vi "labview project submission.vi"() -> ()   [LabVIEW 2012]
uses:
  <vilib>/DAQmx/read.llb/DAQmx Read (Counter DBL 1Chan 1Samp).vi
  <vilib>/DAQmx/write.llb/DAQmx Write (Analog DBL 1Chan 1Samp).vi
  <vilib>/DAQmx/write.llb/DAQmx Write (Digital U8 1Chan 1Samp).vi
  <vilib>/DAQmx/write.llb/DAQmx Write (Digital 1D Bool NChan 1Samp 1Line).vi
  <vilib>/DAQmx/read.llb/DAQmx Read (Analog DBL 1Chan 1Samp).vi
  <vilib>/DAQmx/create/channels.llb/DAQmx Create Channel (CI-Count Edges).vi
  <vilib>/DAQmx/create/channels.llb/DAQmx Create Channel (DO-Digital Output).vi
  <vilib>/DAQmx/create/channels.llb/DAQmx Create Channel (AI-Voltage-Basic).vi
  <vilib>/DAQmx/create/channels.llb/DAQmx Create Channel (AO-Voltage-Basic).vi
  <vilib>/DAQmx/miscellaneous.llb/DAQmx Fill In Error Info.vi
  KERNEL32.DLL
panel:
  out "led 3":bool
  out "led 1":bool
  out "led 2":bool
  out "7 Segment":picture
  out "Voltage:":dbl
  out "Slot Count:":dbl
  out "Data to Write":u32=255 caption="Data to Write:" format="%x"
  out "Motor:":bool[](array[boolean])
  out "Time:":string
  out "Date:":string
  in  "Dignostic":bool
  in  "?":bool
  # "Lighthouse Monitoring & Control System"
  # "Normal Mode"
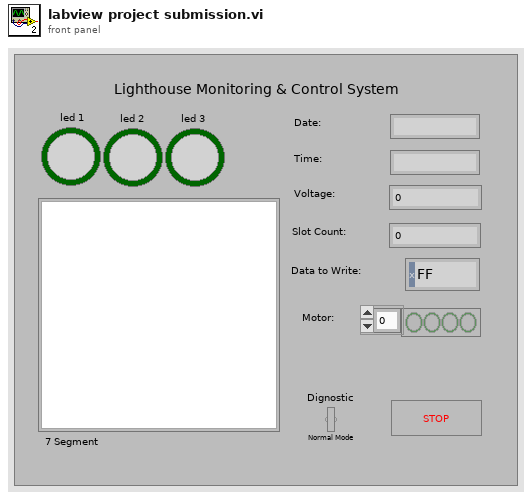
[diagram p1: front panel]
types:
  T1 = typedef "imagedata.ctl" = cluster{"image type":i32, "image depth":i32, "image":u8[], "mask":u8[], "colors":u32[], "Rectangle":cluster{"left":i16, "top":i16, "right":i16, "bottom":i16}}
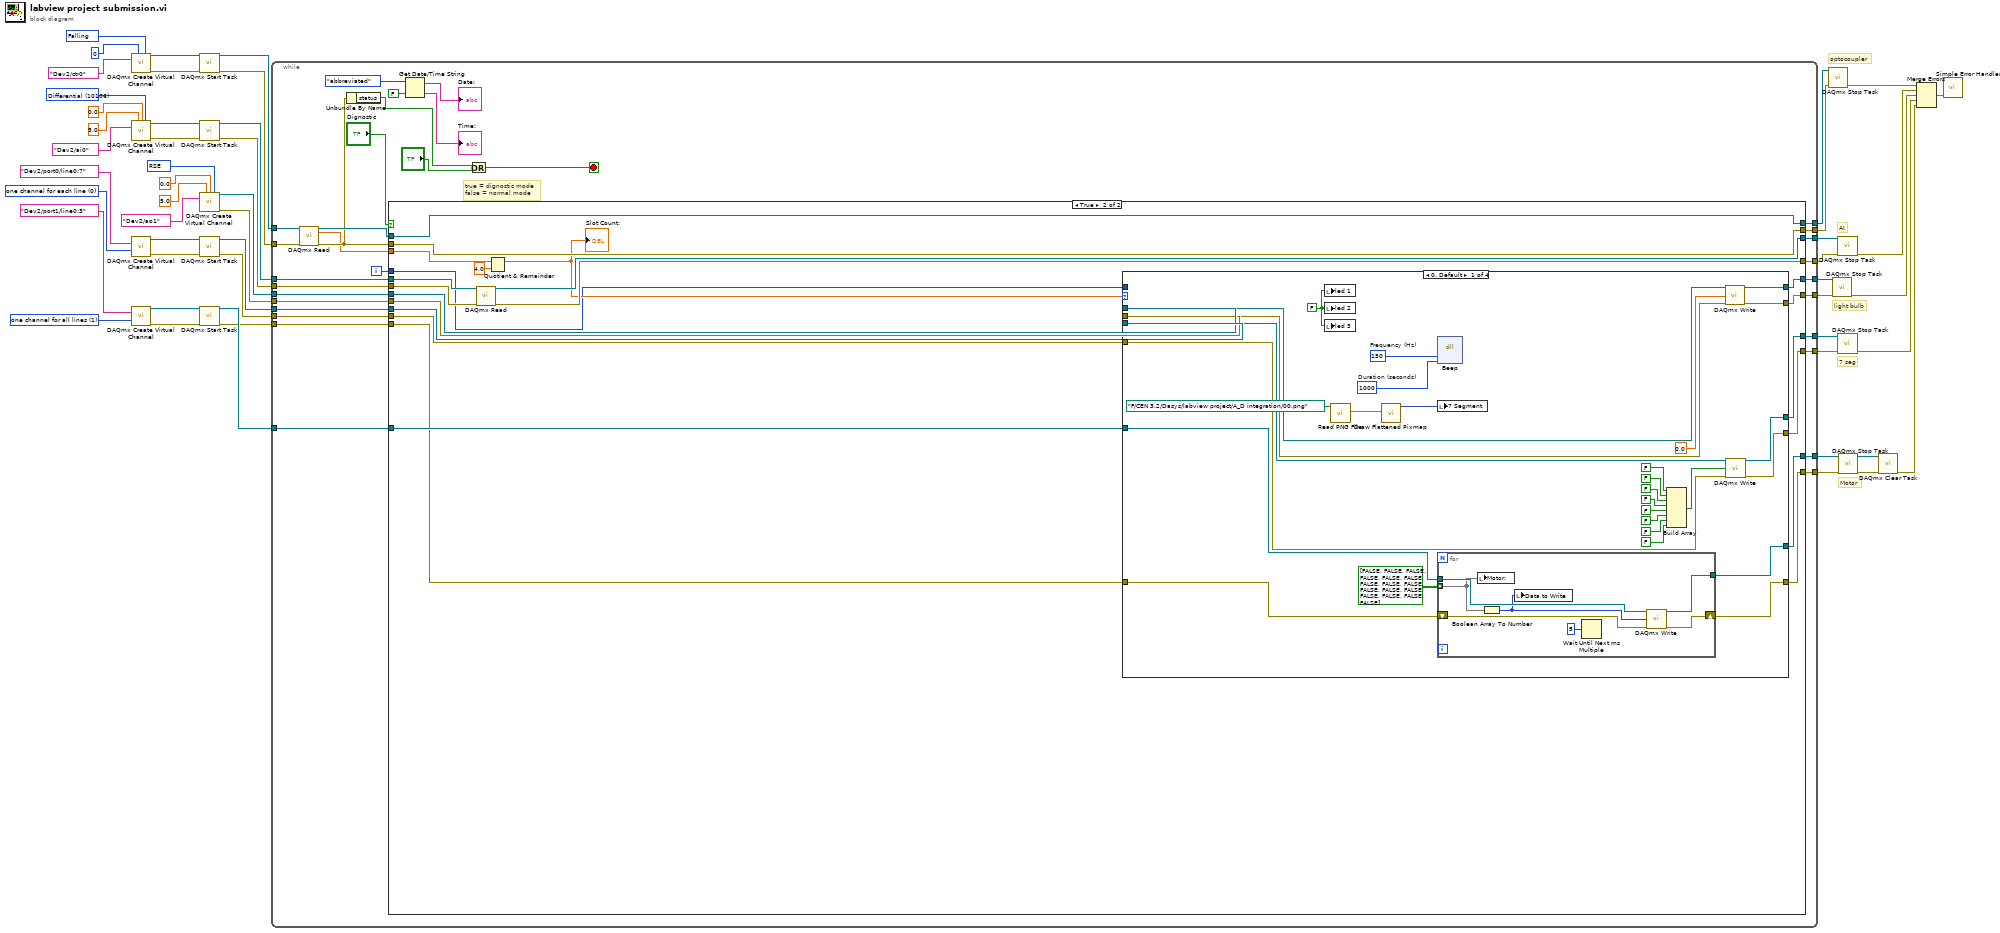
[diagram p0: block diagram]
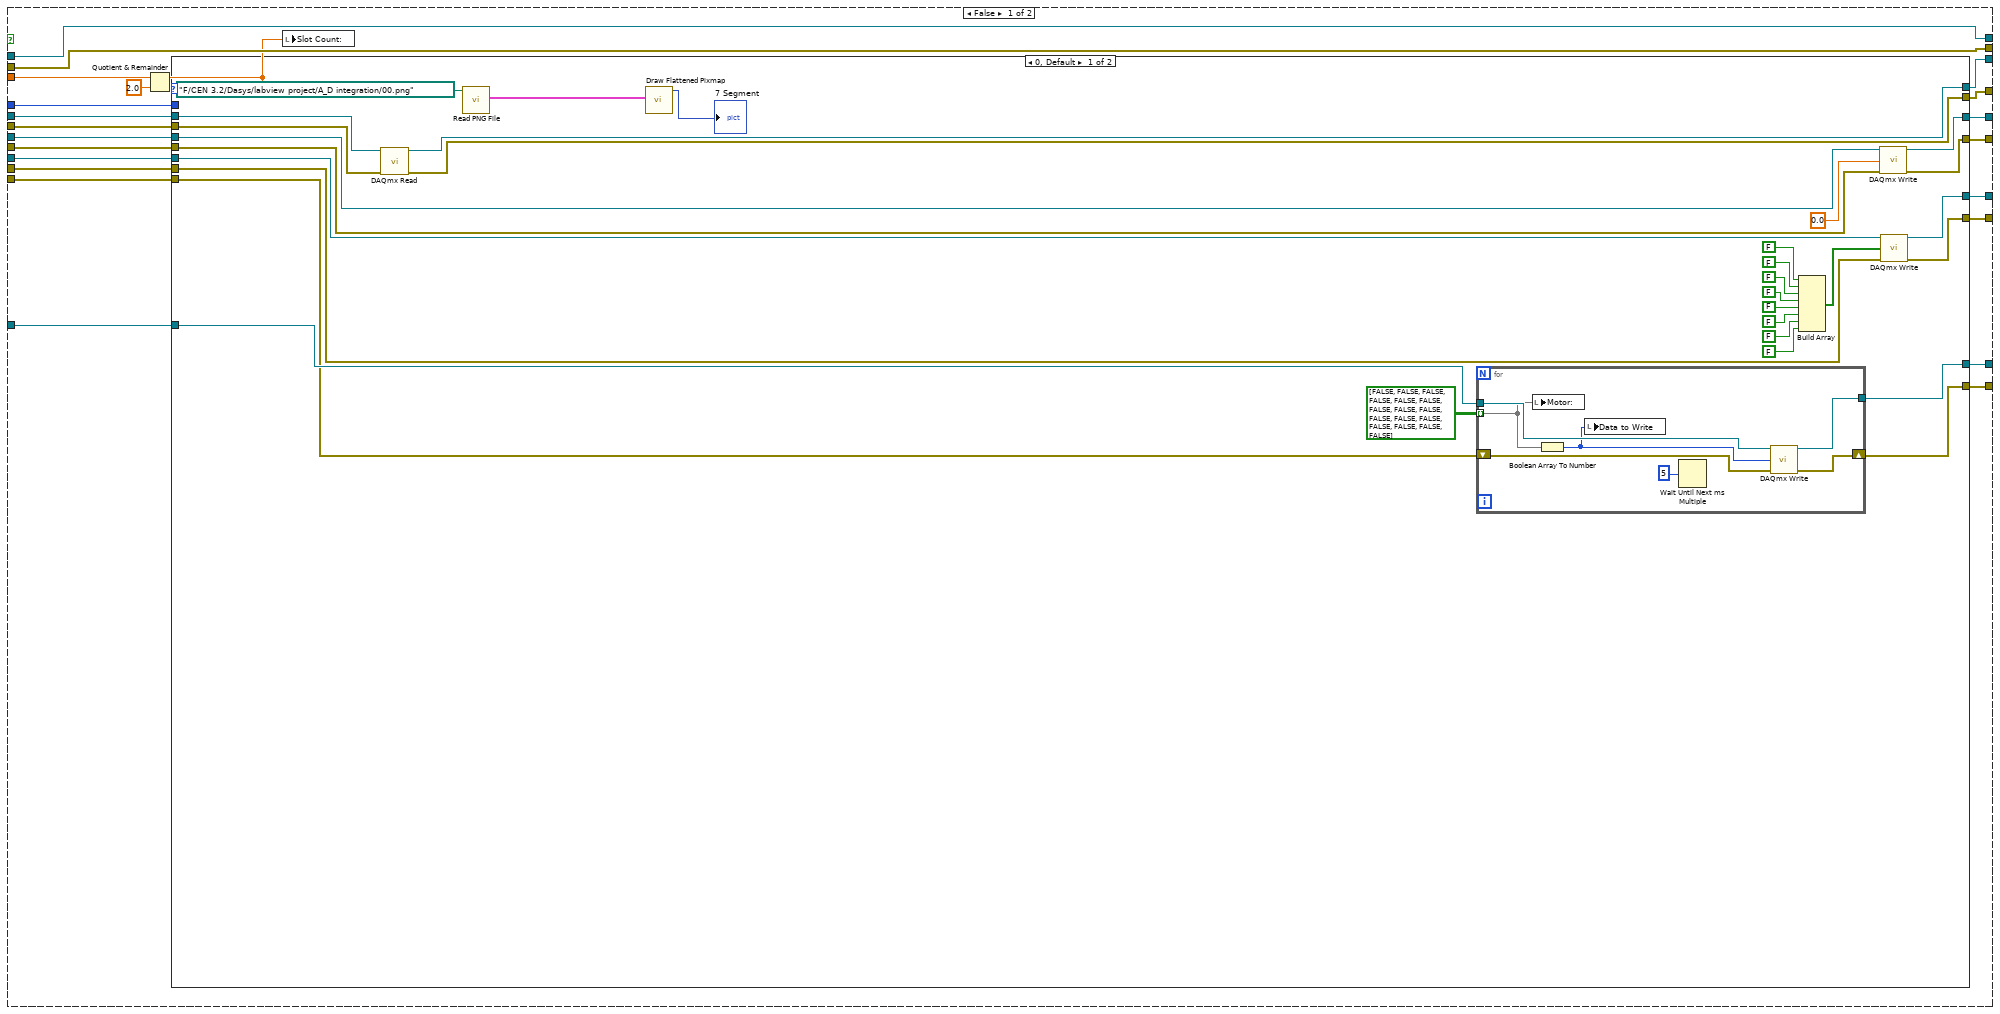
[diagram p2: hidden frame]
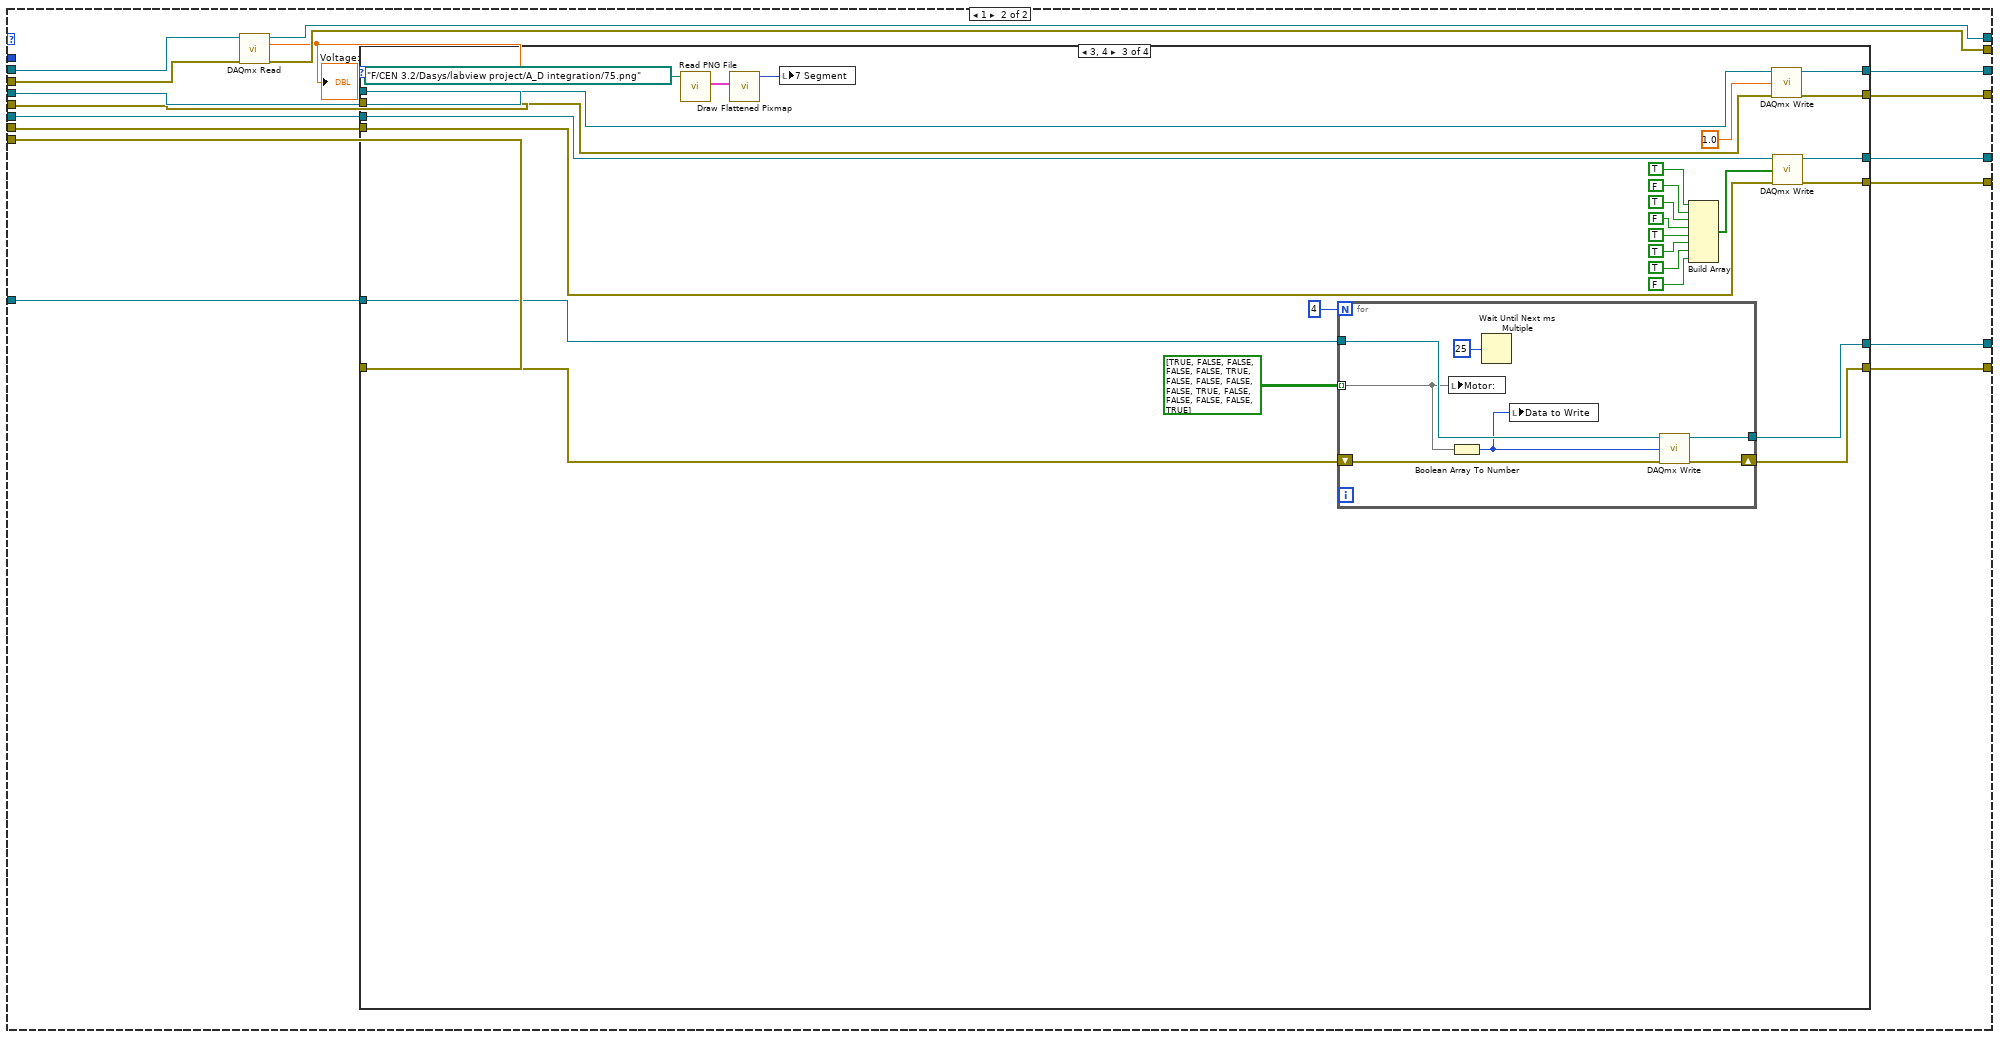
[diagram p3: hidden frame]
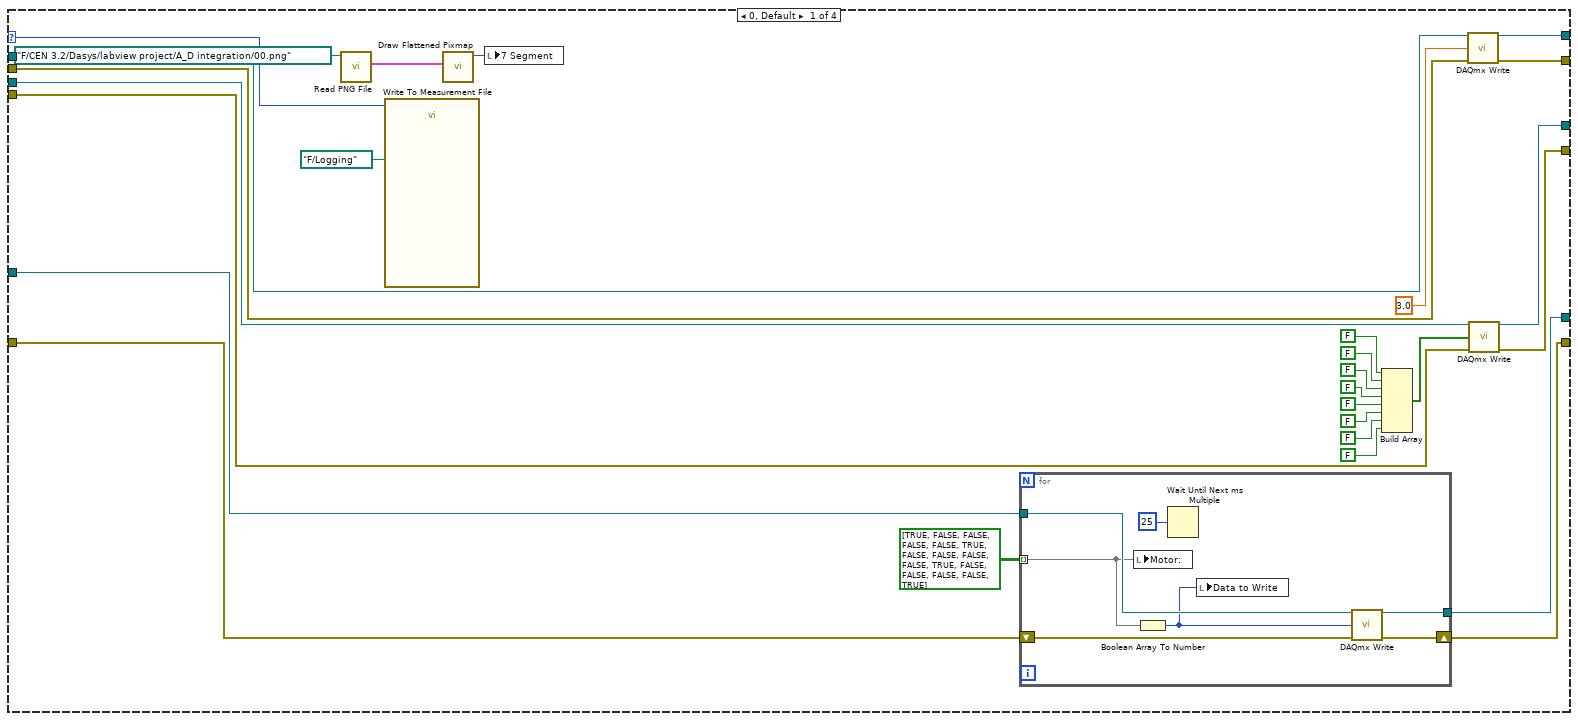
[diagram p4: hidden frame]
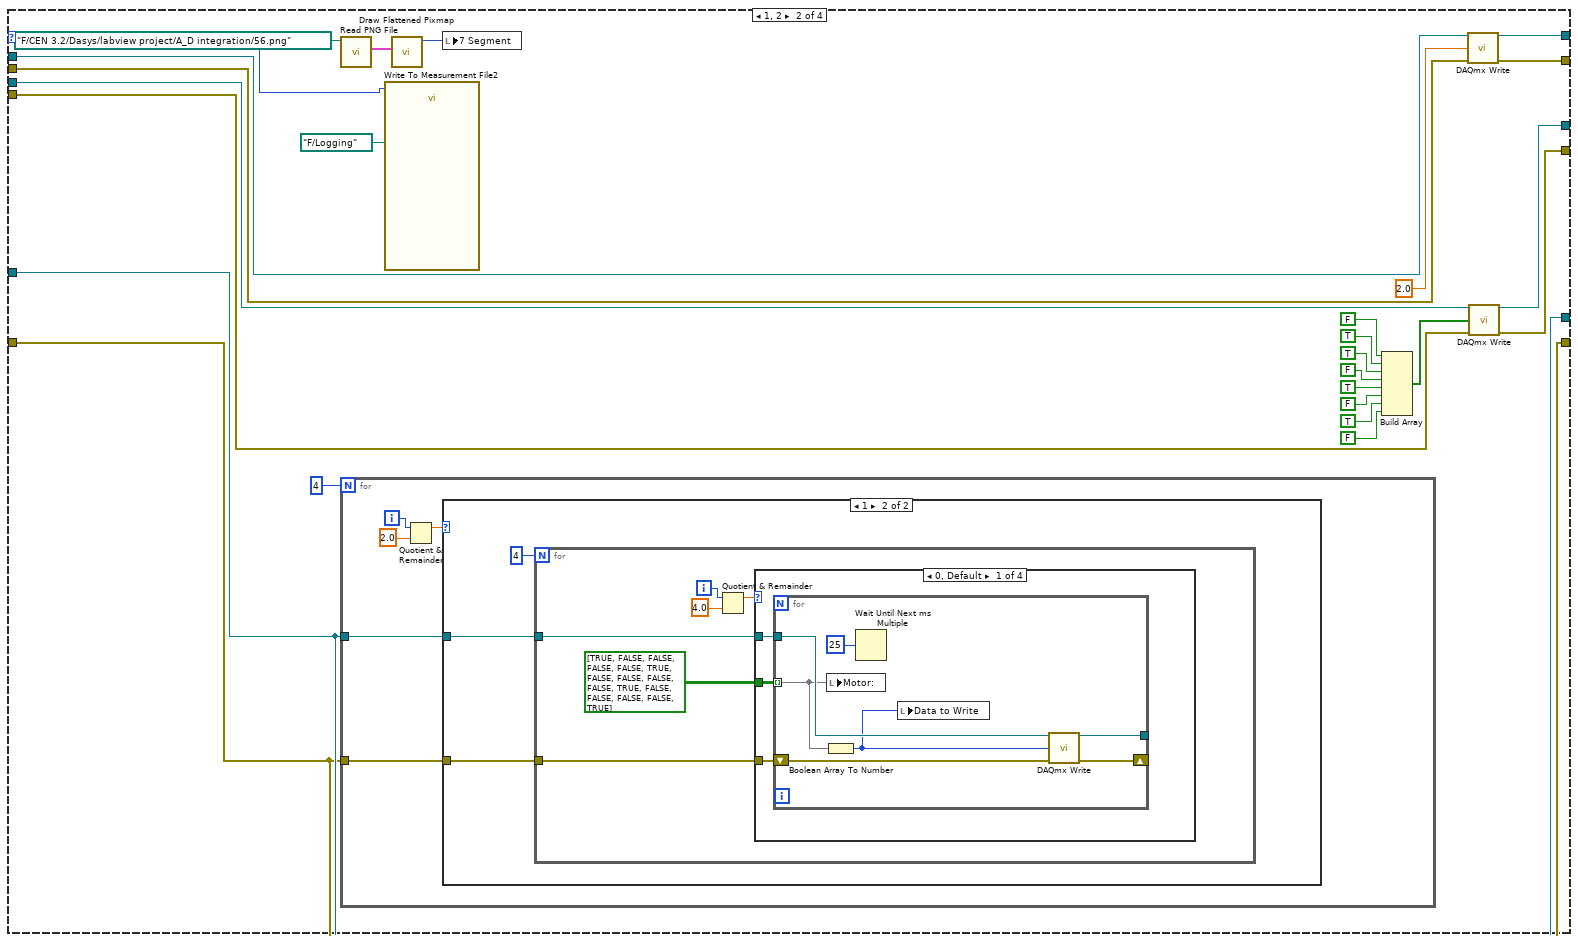
[diagram p5: hidden frame]
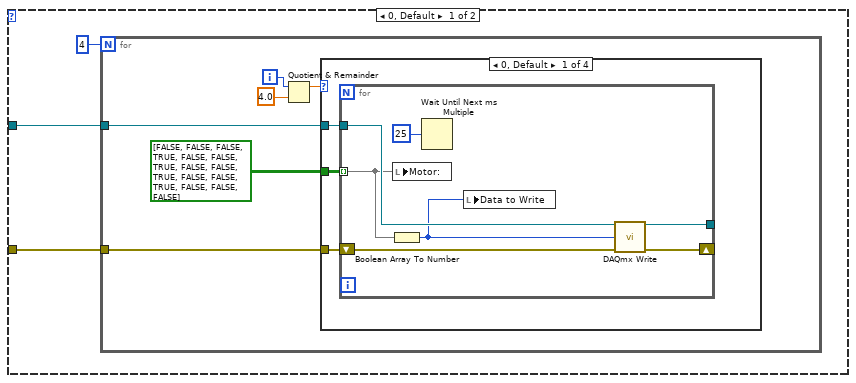
[diagram p6: hidden frame]
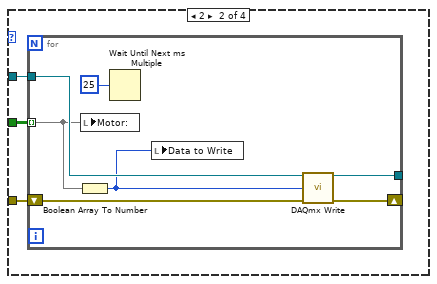
[diagram p7: hidden frame]
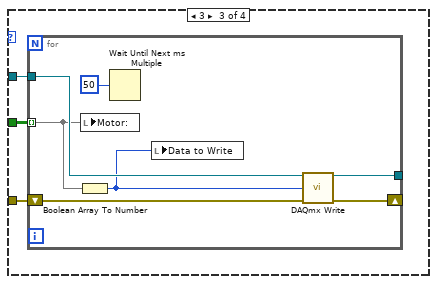
[diagram p8: hidden frame]
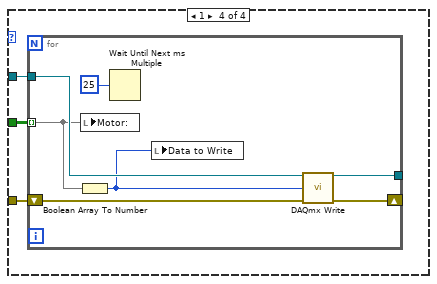
[diagram p9: hidden frame]
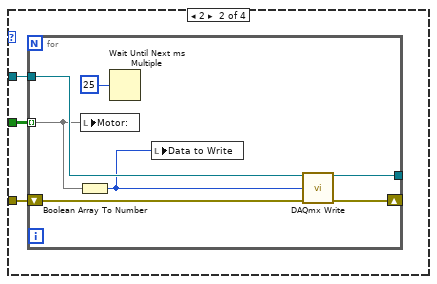
[diagram p10: hidden frame]
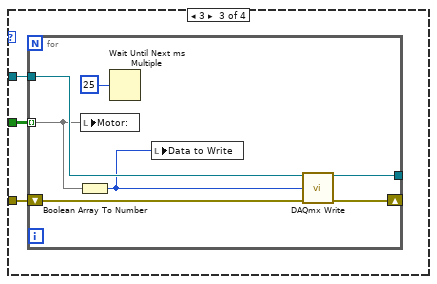
[diagram p11: hidden frame]
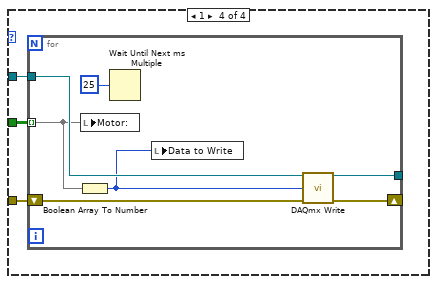
[diagram p12: hidden frame]
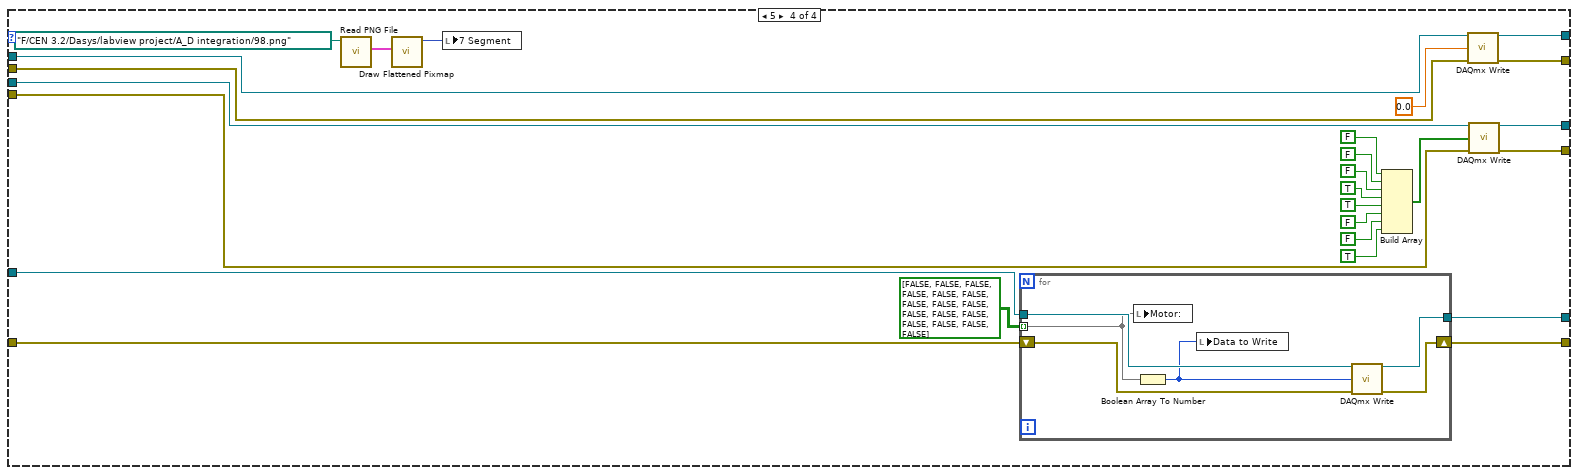
[diagram p13: hidden frame]
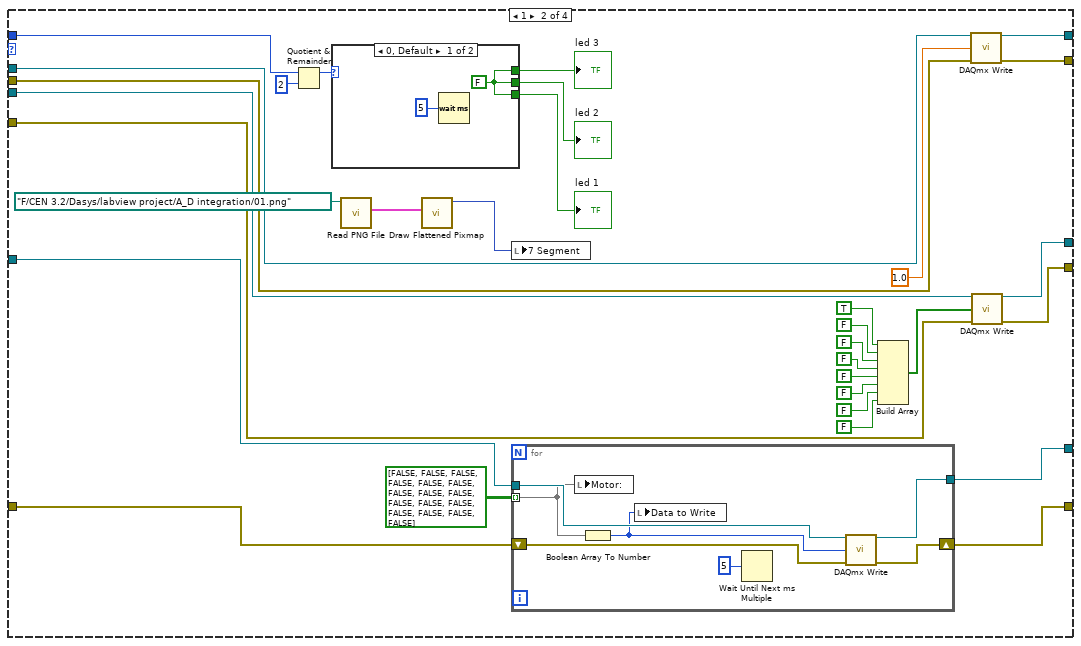
[diagram p14: hidden frame]
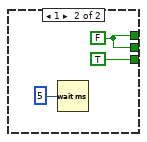
[diagram p15: hidden frame]
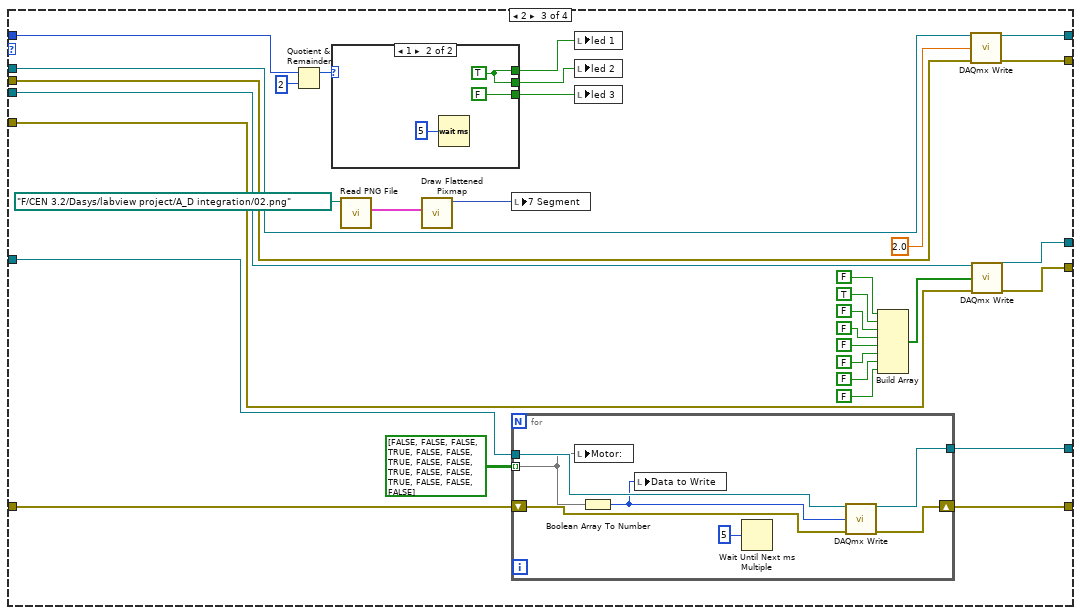
[diagram p16: hidden frame]
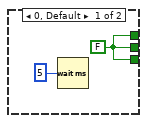
[diagram p17: hidden frame]
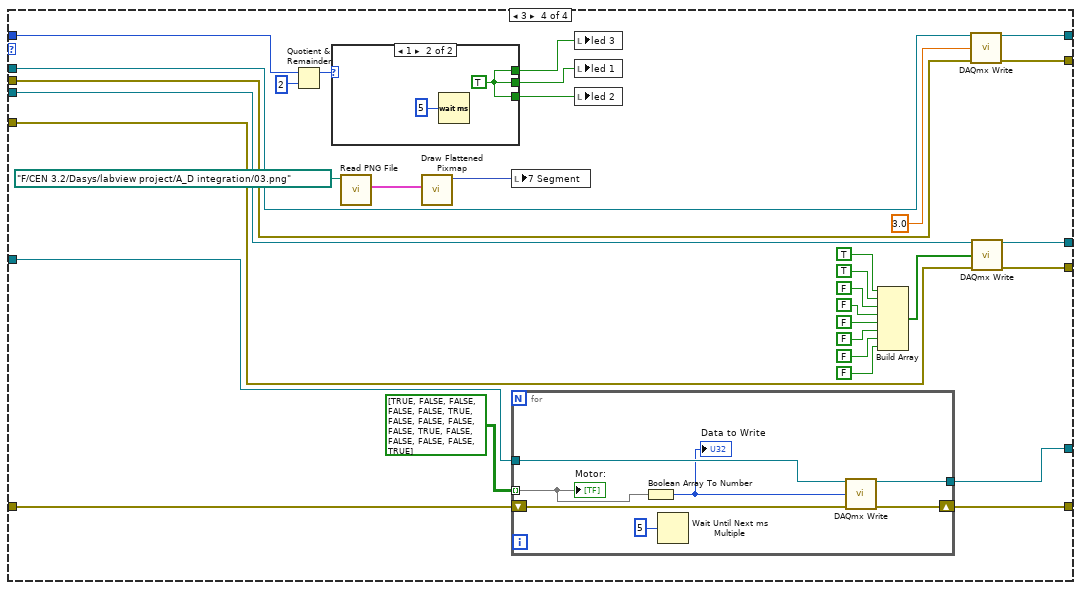
[diagram p18: hidden frame]
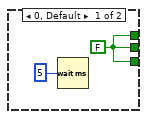
[diagram p19: hidden frame]
diagram:
  w24 = 10083 items=["Default"=-1, "RSE"=10083, "Differential"=10106, "Pseudodifferential"=12529] ("output terminal configuration")
  w32 = 10106 items=["default"=-1, "RSE"=10083, "NRSE"=10078, "Differential"=10106, "Pseudodifferential"=12529] ("input terminal configuration")
  w42 = 1 items=["one channel for each line", "one channel for all lines"] ("line grouping")
  w37 = 0 items=["one channel for each line", "one channel for all lines"] ("line grouping")
  w51 = 10171 items=["Rising"=10280, "Falling"=10171] ("edge")
  # "Motor"
  # "7 seg"
  # "AI"
  # "light bulb"
  # "optocoupler"
  n1 = call-poly <vilib>:"DAQmx Create Virtual Channel.vi"("initial count"=u32 0, "edge"=w51, "counter"=tag "Dev2/ctr0") -> ("task out"=w50:refnum<k21>, "error out"=w49:errorcluster)  [unwired: 11 in]
  n2 = call-poly <vilib>:"DAQmx Create Virtual Channel.vi"("maximum value"=5.0, "minimum value"=0.0, "input terminal configuration"=w32, "physical channels"=tag "Dev2/ai0") -> ("task out"=w30:refnum<k21>, "error out"=w31:errorcluster)  [unwired: 10 in]
  n3 = call-poly <vilib>:"DAQmx Create Virtual Channel.vi"("lines"=tag "Dev2/port0/line0:7", "line grouping"=w37) -> ("task out"=w44:refnum<k21>, "error out"=w43:errorcluster)  [unwired: 12 in]
  n4 = call-poly <vilib>:"DAQmx Create Virtual Channel.vi"("lines"=tag "Dev2/port1/line0:3", "line grouping"=w42) -> ("task out"=w41:refnum<k21>, "error out"=w40:errorcluster)  [unwired: 12 in]
  n5 = call <vilib>:"DAQmx Start Task.vi"("task/channels in"=w50, "error in"=w49) -> ("task out"=w46:refnum<k21>, "error out"=w45:errorcluster)  [unwired: 12 in]
  n6 = call <vilib>:"DAQmx Start Task.vi"("task/channels in"=w30, "error in"=w31) -> ("task out"=w26:refnum<k21>, "error out"=w25:errorcluster)  [unwired: 12 in]
  n7 = call-poly <vilib>:"DAQmx Create Virtual Channel.vi"("maximum value"=5.0, "minimum value"=0.0, "output terminal configuration"=w24, "physical channels"=tag "Dev2/ao1") -> ("task out"=w20:refnum<k21>, "error out"=w19:errorcluster)  [unwired: 10 in]
  n8 = call <vilib>:"DAQmx Start Task.vi"("task/channels in"=w44, "error in"=w43) -> ("task out"=w36:refnum<k21>, "error out"=w35:errorcluster)  [unwired: 12 in]
  n9 = call <vilib>:"DAQmx Start Task.vi"("task/channels in"=w41, "error in"=w40) -> ("task out"=w34:refnum<k21>, "error out"=w33:errorcluster)  [unwired: 12 in]
  n10 = while {
    tunnel: w46 -> [w82]
    tunnel: w45 -> [w81]
    tunnel: w36 -> [w80]
    tunnel: w35 -> [w79]
    tunnel: w34 -> [w78]
    tunnel: w33 -> [w77]
    tunnel: w26 -> [w75]
    tunnel: w25 -> [w74]
    tunnel: w20 -> [w73]
    tunnel: w19 -> [w72]
    tunnel: [w66] -> w10
    tunnel: [w65] -> w9
    tunnel: [w64] -> w8
    tunnel: [w63] -> w7
    tunnel: [w62] -> w6
    tunnel: [w61] -> w5
    tunnel: [w60] -> w4
    tunnel: [w59] -> w3
    tunnel: [w58] -> w2
    tunnel: [w57] -> w1
    i -> [w52]
    stop <- w67 stop-if-true
    # "true = dignostic mode\nfalse = normal mode"
    n11 = call-poly <vilib>:"DAQmx Read.vi"("task/channels in"=w82, "error in"=w81) -> ("task out"=w70:refnum<k21>, "data"=w68:dbl, "error out"=w69:errorcluster)  [unwired: 11 in]
    n12 = Unbundle By Name(w69) -> ("status"=w76:bool)
    n13 = case shown="True" "Dignostic" {
      tunnel: w80 -> [w93 w411]
      tunnel: w79 -> [w92 w410]
      tunnel: w78 -> [w91 w409]
      tunnel: w77 -> [w90 w408]
      tunnel: [w89 w407] -> w60
      tunnel: [w88 w406] -> w59
      tunnel: w75 -> [w103 w403]
      tunnel: w74 -> [w102 w402]
      tunnel: w73 -> [w87 w405]
      tunnel: w72 -> [w86 w404]
      tunnel: [w101 w401] -> w58
      tunnel: [w100 w400] -> w57
      tunnel: [w99 w399] -> w64
      tunnel: [w98 w398] -> w63
      tunnel: [w95 w397] -> w61
      tunnel: [w94 w396] -> w62
      tunnel: w70 -> [w97 w393]
      tunnel: w69 -> [w96 w392]
      tunnel: w68 -> [w104 w394]
      tunnel: [w97 w393] -> w66
      tunnel: [w96 w392] -> w65
      tunnel: w52 -> [w85 w390]
      frame False {
        n14 = Quotient & Remainder(x=w104, y=2.0) -> (x-y*floor(x/y)=w84:dbl)  [unwired: 1 out]
        n15 = case shown="0, Default" w84 {
          tunnel: w103 -> [w134 w159]
          tunnel: w102 -> [w133 w158]
          tunnel: [w130 w157] -> w99
          tunnel: [w131 w156] -> w98
          tunnel: [w132 w155] -> w100
          tunnel: [w127 w154] -> w95
          tunnel: [w128 w153] -> w94
          tunnel: [w129 w152] -> w101
          tunnel: [w115 w150] -> w88
          tunnel: [w116 w151] -> w89
          tunnel: w93 -> [w114 w144]
          tunnel: w92 -> [w113 w143]
          tunnel: w91 -> [w112 w146]
          tunnel: w90 -> [w111 w145]
          tunnel: w87 -> [w110 w148]
          tunnel: w86 -> [w109 w147]
          tunnel: w85 -> [_ _]
          frame 0, Default {
            n16 = call-poly <vilib>:"DAQmx Read.vi"("task/channels in"=w134, "error in"=w133) -> ("task out"=w129:refnum<k21>, "error out"=w132:errorcluster)  [unwired: 11 in, 1 out]
            n17 = call <vilib>:"Read PNG File.vi"("path to PNG file"=path "F:/CEN 3.2/Dasys/labview project/A_D integration/00.png") -> ("image data"=w108:T1)  [unwired: 8 in, 2 out]
            n18 = call <vilib>:"Draw Flattened Pixmap.vi"("image data"=w108) -> ("new picture"=→"7 Segment":picture)  [unwired: 8 in]
            n19 = for {
              tunnel: [w141] -> w116
              shift-right: [w139] -> w115
              shift-left: w111 -> [w142]
              tunnel: bool[][] [[FALSE, FALSE, FALSE, FALSE], [FALSE, FALSE, FALSE, FALSE], [FALSE, FALSE, FALSE, FALSE], [FALSE, FALSE, FALSE, FALSE]] -> [w136] mode=indexing
              tunnel: w112 -> [w138]
              n20 = local write "Motor:"(w136) -> ()
              n21 = Boolean Array To Number(Boolean array=w136) -> (number=w137:u32)
              n22 = local write "Data to Write"(w137) -> ()
              n23 = Wait Until Next ms Multiple(millisecond multiple=5) -> ()  [unwired: 1 out]
              n24 = call-poly <vilib>:"DAQmx Write.vi"("task/channels in"=w138, "data"=w137, "error in"=w142) -> ("task out"=w141:refnum<k21>, "error out"=w139:errorcluster)  [unwired: 10 in, 1 out]
            }
            n25 = Build Array(FALSE, FALSE, FALSE, FALSE, FALSE, FALSE, FALSE, FALSE) -> (w118:bool[])
            n26 = call-poly <vilib>:"DAQmx Write.vi"("task/channels in"=w110, "data"=0.0, "error in"=w109) -> ("task out"=w130:refnum<k21>, "error out"=w131:errorcluster)  [unwired: 10 in, 1 out]
            n27 = call-poly <vilib>:"DAQmx Write.vi"("task/channels in"=w114, "data"=w118, "error in"=w113) -> ("task out"=w128:refnum<k21>, "error out"=w127:errorcluster)  [unwired: 10 in, 1 out]
          }
          frame 1 {
            n28 = call-poly <vilib>:"DAQmx Read.vi"("task/channels in"=w159, "error in"=w158) -> ("task out"=w152:refnum<k21>, "data"=w149:dbl, "error out"=w155:errorcluster)  [unwired: 11 in]
            "Voltage:" <- w149
            n29 = case shown="3, 4" w149 {
              selector: w149 -> [w169 w205 _ _]
              tunnel: [w177 w210 w340 w373] -> w157
              tunnel: [w176 w209 w339 w372] -> w156
              tunnel: [w175 w208 w338 w371] -> w153
              tunnel: [w174 w207 w337 w370] -> w154
              tunnel: [w173 w199 w335 w368] -> w151
              tunnel: [w172 w198 w334 w367] -> w150
              tunnel: w148 -> [w168 w204 w333 w366]
              tunnel: w147 -> [w167 w203 w332 w365]
              tunnel: w146 -> [w166 w199 w329 w362]
              tunnel: w145 -> [w163 w198 w328 w361]
              tunnel: w144 -> [w165 w202 w331 w364]
              tunnel: w143 -> [w164 w201 w330 w363]
              frame 0, Default {
                n30 = call <vilib>:"Read PNG File.vi"("path to PNG file"=path "F:/CEN 3.2/Dasys/labview project/A_D integration/00.png") -> ("image data"=w162:T1)  [unwired: 8 in, 2 out]
                n31 = call "Write To Measurement File"("Signals"=w169, "Filename"=path "F:/Logging") -> ()  [unwired: 15 in, 3 out]
                n32 = call <vilib>:"Draw Flattened Pixmap.vi"("image data"=w162) -> ("new picture"=w161:picture)  [unwired: 8 in]
                n33 = local write "7 Segment"(w161) -> ()
                n34 = for {
                  tunnel: [w193] -> w173
                  shift-right: [w192] -> w172
                  shift-left: w163 -> [w194]
                  tunnel: bool[][] [[TRUE, FALSE, FALSE, FALSE], [FALSE, TRUE, FALSE, FALSE], [FALSE, FALSE, TRUE, FALSE], [FALSE, FALSE, FALSE, TRUE]] -> [w188] mode=indexing
                  tunnel: w166 -> [w190]
                  n35 = local write "Motor:"(w188) -> ()
                  n36 = Boolean Array To Number(Boolean array=w188) -> (number=w189:u32)
                  n37 = Wait Until Next ms Multiple(millisecond multiple=u32 25) -> ()  [unwired: 1 out]
                  n38 = local write "Data to Write"(w189) -> ()
                  n39 = call-poly <vilib>:"DAQmx Write.vi"("task/channels in"=w190, "data"=w189, "error in"=w194) -> ("task out"=w193:refnum<k21>, "error out"=w192:errorcluster)  [unwired: 10 in, 1 out]
                }
                n40 = Build Array(FALSE, FALSE, FALSE, FALSE, FALSE, FALSE, FALSE, FALSE) -> (w178:bool[])
                n41 = call-poly <vilib>:"DAQmx Write.vi"("task/channels in"=w168, "data"=3.0, "error in"=w167) -> ("task out"=w177:refnum<k21>, "error out"=w176:errorcluster)  [unwired: 10 in, 1 out]
                n42 = call-poly <vilib>:"DAQmx Write.vi"("task/channels in"=w165, "data"=w178, "error in"=w164) -> ("task out"=w175:refnum<k21>, "error out"=w174:errorcluster)  [unwired: 10 in, 1 out]
              }
              frame 1, 2 {
                n43 = call <vilib>:"Read PNG File.vi"("path to PNG file"=path "F:/CEN 3.2/Dasys/labview project/A_D integration/56.png") -> ("image data"=w197:T1)  [unwired: 8 in, 2 out]
                n44 = for {
                  N: 4 -> [_]
                  tunnel: w199 -> [w225]
                  tunnel: w198 -> [w224]
                  i -> [w222]
                  n45 = Quotient & Remainder(x=w222, y=2.0) -> (x-y*floor(x/y)=w221:dbl)  [unwired: 1 out]
                  n46 = case shown="1" w221 {
                    tunnel: w225 -> [w228 w277]
                    tunnel: w224 -> [w227 w276]
                    frame 0, Default {
                      n47 = for {
                        N: 4 -> [_]
                        tunnel: w228 -> [w234]
                        tunnel: w227 -> [w233]
                        i -> [w230]
                        n48 = Quotient & Remainder(x=w230, y=4.0) -> (x-y*floor(x/y)=w229:dbl)  [unwired: 1 out]
                        n49 = case shown="0, Default" w229 {
                          tunnel: w234 -> [w237 w247 w256 w267]
                          tunnel: w233 -> [w235 w246 w257 w266]
                          tunnel: bool[][] [[FALSE, FALSE, FALSE, TRUE], [FALSE, FALSE, TRUE, FALSE], [FALSE, TRUE, FALSE, FALSE], [TRUE, FALSE, FALSE, FALSE]] -> [w236 w245 w255 w265]
                          frame 0, Default {
                            n50 = for {
                              tunnel: [w243] -> _
                              shift-right: [w242] -> _
                              shift-left: w235 -> [w244]
                              tunnel: w236 -> [w238] mode=indexing
                              tunnel: w237 -> [w240]
                              n51 = Boolean Array To Number(Boolean array=w238) -> (number=w239:u32)
                              n52 = local write "Motor:"(w238) -> ()
                              n53 = Wait Until Next ms Multiple(millisecond multiple=u32 25) -> ()  [unwired: 1 out]
                              n54 = local write "Data to Write"(w239) -> ()
                              n55 = call-poly <vilib>:"DAQmx Write.vi"("task/channels in"=w240, "data"=w239, "error in"=w244) -> ("task out"=w243:refnum<k21>, "error out"=w242:errorcluster)  [unwired: 10 in, 1 out]
                            }
                          }
                          frame 2 {
                            n56 = for {
                              tunnel: [w253] -> _
                              shift-right: [w252] -> _
                              shift-left: w246 -> [w254]
                              tunnel: w245 -> [w248] mode=indexing
                              tunnel: w247 -> [w250]
                              n57 = Boolean Array To Number(Boolean array=w248) -> (number=w249:u32)
                              n58 = local write "Motor:"(w248) -> ()
                              n59 = Wait Until Next ms Multiple(millisecond multiple=u32 25) -> ()  [unwired: 1 out]
                              n60 = local write "Data to Write"(w249) -> ()
                              n61 = call-poly <vilib>:"DAQmx Write.vi"("task/channels in"=w250, "data"=w249, "error in"=w254) -> ("task out"=w253:refnum<k21>, "error out"=w252:errorcluster)  [unwired: 10 in, 1 out]
                            }
                          }
                          frame 3 {
                            n62 = for {
                              tunnel: [w263] -> _
                              shift-right: [w262] -> _
                              shift-left: w257 -> [w264]
                              tunnel: w255 -> [w259] mode=indexing
                              tunnel: w256 -> [w260]
                              n63 = Boolean Array To Number(Boolean array=w259) -> (number=w258:u32)
                              n64 = local write "Motor:"(w259) -> ()
                              n65 = Wait Until Next ms Multiple(millisecond multiple=u32 50) -> ()  [unwired: 1 out]
                              n66 = local write "Data to Write"(w258) -> ()
                              n67 = call-poly <vilib>:"DAQmx Write.vi"("task/channels in"=w260, "data"=w258, "error in"=w264) -> ("task out"=w263:refnum<k21>, "error out"=w262:errorcluster)  [unwired: 10 in, 1 out]
                            }
                          }
                          frame 1 {
                            n68 = for {
                              tunnel: [w273] -> _
                              shift-right: [w272] -> _
                              shift-left: w266 -> [w274]
                              tunnel: w265 -> [w269] mode=indexing
                              tunnel: w267 -> [w270]
                              n69 = Boolean Array To Number(Boolean array=w269) -> (number=w268:u32)
                              n70 = local write "Motor:"(w269) -> ()
                              n71 = Wait Until Next ms Multiple(millisecond multiple=u32 25) -> ()  [unwired: 1 out]
                              n72 = local write "Data to Write"(w268) -> ()
                              n73 = call-poly <vilib>:"DAQmx Write.vi"("task/channels in"=w270, "data"=w268, "error in"=w274) -> ("task out"=w273:refnum<k21>, "error out"=w272:errorcluster)  [unwired: 10 in, 1 out]
                            }
                          }
                        }
                      }
                    }
                    frame 1 {
                      n74 = for {
                        N: 4 -> [_]
                        tunnel: w277 -> [w283]
                        tunnel: w276 -> [w282]
                        i -> [w281]
                        n75 = Quotient & Remainder(x=w281, y=4.0) -> (x-y*floor(x/y)=w279:dbl)  [unwired: 1 out]
                        n76 = case shown="0, Default" w279 {
                          tunnel: w283 -> [w286 w296 w305 w316]
                          tunnel: w282 -> [w285 w295 w306 w315]
                          tunnel: bool[][] [[TRUE, FALSE, FALSE, FALSE], [FALSE, TRUE, FALSE, FALSE], [FALSE, FALSE, TRUE, FALSE], [FALSE, FALSE, FALSE, TRUE]] -> [w284 w294 w304 w314]
                          frame 0, Default {
                            n77 = for {
                              tunnel: [w292] -> _
                              shift-right: [w291] -> _
                              shift-left: w285 -> [w293]
                              tunnel: w284 -> [w288] mode=indexing
                              tunnel: w286 -> [w289]
                              n78 = Boolean Array To Number(Boolean array=w288) -> (number=w287:u32)
                              n79 = local write "Motor:"(w288) -> ()
                              n80 = Wait Until Next ms Multiple(millisecond multiple=u32 25) -> ()  [unwired: 1 out]
                              n81 = local write "Data to Write"(w287) -> ()
                              n82 = call-poly <vilib>:"DAQmx Write.vi"("task/channels in"=w289, "data"=w287, "error in"=w293) -> ("task out"=w292:refnum<k21>, "error out"=w291:errorcluster)  [unwired: 10 in, 1 out]
                            }
                          }
                          frame 2 {
                            n83 = for {
                              tunnel: [w302] -> _
                              shift-right: [w301] -> _
                              shift-left: w295 -> [w303]
                              tunnel: w294 -> [w297] mode=indexing
                              tunnel: w296 -> [w299]
                              n84 = Boolean Array To Number(Boolean array=w297) -> (number=w298:u32)
                              n85 = local write "Motor:"(w297) -> ()
                              n86 = Wait Until Next ms Multiple(millisecond multiple=u32 25) -> ()  [unwired: 1 out]
                              n87 = local write "Data to Write"(w298) -> ()
                              n88 = call-poly <vilib>:"DAQmx Write.vi"("task/channels in"=w299, "data"=w298, "error in"=w303) -> ("task out"=w302:refnum<k21>, "error out"=w301:errorcluster)  [unwired: 10 in, 1 out]
                            }
                          }
                          frame 3 {
                            n89 = for {
                              tunnel: [w312] -> _
                              shift-right: [w311] -> _
                              shift-left: w306 -> [w313]
                              tunnel: w304 -> [w308] mode=indexing
                              tunnel: w305 -> [w309]
                              n90 = Boolean Array To Number(Boolean array=w308) -> (number=w307:u32)
                              n91 = local write "Motor:"(w308) -> ()
                              n92 = Wait Until Next ms Multiple(millisecond multiple=u32 25) -> ()  [unwired: 1 out]
                              n93 = local write "Data to Write"(w307) -> ()
                              n94 = call-poly <vilib>:"DAQmx Write.vi"("task/channels in"=w309, "data"=w307, "error in"=w313) -> ("task out"=w312:refnum<k21>, "error out"=w311:errorcluster)  [unwired: 10 in, 1 out]
                            }
                          }
                          frame 1 {
                            n95 = for {
                              tunnel: [w322] -> _
                              shift-right: [w321] -> _
                              shift-left: w315 -> [w323]
                              tunnel: w314 -> [w318] mode=indexing
                              tunnel: w316 -> [w319]
                              n96 = Boolean Array To Number(Boolean array=w318) -> (number=w317:u32)
                              n97 = local write "Motor:"(w318) -> ()
                              n98 = Wait Until Next ms Multiple(millisecond multiple=u32 25) -> ()  [unwired: 1 out]
                              n99 = local write "Data to Write"(w317) -> ()
                              n100 = call-poly <vilib>:"DAQmx Write.vi"("task/channels in"=w319, "data"=w317, "error in"=w323) -> ("task out"=w322:refnum<k21>, "error out"=w321:errorcluster)  [unwired: 10 in, 1 out]
                            }
                          }
                        }
                      }
                    }
                  }
                }
                n101 = call "Write To Measurement File2"("Signals"=w205, "Filename"=path "F:/Logging") -> ()  [unwired: 15 in, 3 out]
                n102 = call <vilib>:"Draw Flattened Pixmap.vi"("image data"=w197) -> ("new picture"=w196:picture)  [unwired: 8 in]
                n103 = local write "7 Segment"(w196) -> ()
                n104 = Build Array(FALSE, TRUE, TRUE, FALSE, TRUE, FALSE, TRUE, FALSE) -> (w211:bool[])
                n105 = call-poly <vilib>:"DAQmx Write.vi"("task/channels in"=w204, "data"=2.0, "error in"=w203) -> ("task out"=w210:refnum<k21>, "error out"=w209:errorcluster)  [unwired: 10 in, 1 out]
                n106 = call-poly <vilib>:"DAQmx Write.vi"("task/channels in"=w202, "data"=w211, "error in"=w201) -> ("task out"=w208:refnum<k21>, "error out"=w207:errorcluster)  [unwired: 10 in, 1 out]
              }
              frame 3, 4 {
                n107 = call <vilib>:"Read PNG File.vi"("path to PNG file"=path "F:/CEN 3.2/Dasys/labview project/A_D integration/75.png") -> ("image data"=w326:T1)  [unwired: 8 in, 2 out]
                n108 = call <vilib>:"Draw Flattened Pixmap.vi"("image data"=w326) -> ("new picture"=w325:picture)  [unwired: 8 in]
                n109 = local write "7 Segment"(w325) -> ()
                n110 = for {
                  N: 4 -> [_]
                  tunnel: [w356] -> w335
                  shift-right: [w355] -> w334
                  shift-left: w328 -> [w357]
                  tunnel: bool[][] [[TRUE, FALSE, FALSE, FALSE], [FALSE, TRUE, FALSE, FALSE], [FALSE, FALSE, TRUE, FALSE], [FALSE, FALSE, FALSE, TRUE]] -> [w352] mode=indexing
                  tunnel: w329 -> [w354]
                  n111 = local write "Motor:"(w352) -> ()
                  n112 = Boolean Array To Number(Boolean array=w352) -> (number=w353:u32)
                  n113 = Wait Until Next ms Multiple(millisecond multiple=u32 25) -> ()  [unwired: 1 out]
                  n114 = local write "Data to Write"(w353) -> ()
                  n115 = call-poly <vilib>:"DAQmx Write.vi"("task/channels in"=w354, "data"=w353, "error in"=w357) -> ("task out"=w356:refnum<k21>, "error out"=w355:errorcluster)  [unwired: 10 in, 1 out]
                }
                n116 = Build Array(TRUE, FALSE, TRUE, FALSE, TRUE, TRUE, TRUE, FALSE) -> (w341:bool[])
                n117 = call-poly <vilib>:"DAQmx Write.vi"("task/channels in"=w333, "data"=1.0, "error in"=w332) -> ("task out"=w340:refnum<k21>, "error out"=w339:errorcluster)  [unwired: 10 in, 1 out]
                n118 = call-poly <vilib>:"DAQmx Write.vi"("task/channels in"=w331, "data"=w341, "error in"=w330) -> ("task out"=w338:refnum<k21>, "error out"=w337:errorcluster)  [unwired: 10 in, 1 out]
              }
              frame 5 {
                n119 = call <vilib>:"Read PNG File.vi"("path to PNG file"=path "F:/CEN 3.2/Dasys/labview project/A_D integration/98.png") -> ("image data"=w360:T1)  [unwired: 8 in, 2 out]
                n120 = call <vilib>:"Draw Flattened Pixmap.vi"("image data"=w360) -> ("new picture"=w359:picture)  [unwired: 8 in]
                n121 = local write "7 Segment"(w359) -> ()
                n122 = for {
                  tunnel: [w388] -> w368
                  shift-right: [w387] -> w367
                  shift-left: w361 -> [w389]
                  tunnel: bool[][] [[FALSE, FALSE, FALSE, FALSE], [FALSE, FALSE, FALSE, FALSE], [FALSE, FALSE, FALSE, FALSE], [FALSE, FALSE, FALSE, FALSE]] -> [w384] mode=indexing
                  tunnel: w362 -> [w386]
                  n123 = local write "Motor:"(w384) -> ()
                  n124 = Boolean Array To Number(Boolean array=w384) -> (number=w385:u32)
                  n125 = local write "Data to Write"(w385) -> ()
                  n126 = call-poly <vilib>:"DAQmx Write.vi"("task/channels in"=w386, "data"=w385, "error in"=w389) -> ("task out"=w388:refnum<k21>, "error out"=w387:errorcluster)  [unwired: 10 in, 1 out]
                }
                n127 = Build Array(FALSE, FALSE, FALSE, TRUE, TRUE, FALSE, FALSE, TRUE) -> (w374:bool[])
                n128 = call-poly <vilib>:"DAQmx Write.vi"("task/channels in"=w366, "data"=0.0, "error in"=w365) -> ("task out"=w373:refnum<k21>, "error out"=w372:errorcluster)  [unwired: 10 in, 1 out]
                n129 = call-poly <vilib>:"DAQmx Write.vi"("task/channels in"=w364, "data"=w374, "error in"=w363) -> ("task out"=w371:refnum<k21>, "error out"=w370:errorcluster)  [unwired: 10 in, 1 out]
              }
            }
          }
        }
        n130 = local write "Slot Count:"(w84) -> ()
      }
      frame True {
        n131 = call-poly <vilib>:"DAQmx Read.vi"("task/channels in"=w403, "error in"=w402) -> ("task out"=w401:refnum<k21>, "error out"=w400:errorcluster)  [unwired: 11 in, 1 out]
        n132 = Quotient & Remainder(x=w394, y=4.0) -> (x-y*floor(x/y)=w391:dbl)  [unwired: 1 out]
        "Slot Count:" <- w391
        n133 = case shown="0, Default" w391 {
          tunnel: w411 -> [w428 w465 w509 w552]
          tunnel: w410 -> [w427 w464 w510 w553]
          tunnel: w409 -> [w440 w463 w506 w550]
          tunnel: w408 -> [w439 w462 w507 w549]
          tunnel: [w438 w461 w505 w548] -> w407
          tunnel: [w437 w460 w504 w547] -> w406
          tunnel: w405 -> [w425 w476 w520 w564]
          tunnel: w404 -> [w424 w475 w519 w563]
          tunnel: [w423 w478 w522 w566] -> w399
          tunnel: [w422 w477 w521 w565] -> w398
          tunnel: [w420 w458 w502 w546] -> w396
          tunnel: [w419 w457 w501 w545] -> w397
          tunnel: w390 -> [_ w451 w495 w539]
          frame 0, Default {
            w414 = 150  # Frequency (Hz)
            w413 = 1000  # Duration (seconds)
            w415 = FALSE
            n134 = local write "led 1"(w415) -> ()
            n135 = local write "led 2"(w415) -> ()
            n136 = local write "led 3"(w415) -> ()
            n137 = call <vilib>:"Read PNG File.vi"("path to PNG file"=path "F:/CEN 3.2/Dasys/labview project/A_D integration/00.png") -> ("image data"=w417:T1)  [unwired: 8 in, 2 out]
            n138 = call <vilib>:"Draw Flattened Pixmap.vi"("image data"=w417) -> ("new picture"=w416:picture)  [unwired: 8 in]
            n139 = dll-call lib="KERNEL32.DLL" fn="Beep"(w414, w413) -> ()  [unwired: 6 in, 2 out]
            n140 = local write "7 Segment"(w416) -> ()
            n141 = for {
              tunnel: [w446] -> w438
              shift-right: [w444] -> w437
              shift-left: w439 -> [w447]
              tunnel: w440 -> [w443]
              tunnel: bool[][] [[FALSE, FALSE, FALSE, FALSE], [FALSE, FALSE, FALSE, FALSE], [FALSE, FALSE, FALSE, FALSE], [FALSE, FALSE, FALSE, FALSE]] -> [w441] mode=indexing
              n142 = local write "Motor:"(w441) -> ()
              n143 = Boolean Array To Number(Boolean array=w441) -> (number=w442:u32)
              n144 = local write "Data to Write"(w442) -> ()
              n145 = Wait Until Next ms Multiple(millisecond multiple=5) -> ()  [unwired: 1 out]
              n146 = call-poly <vilib>:"DAQmx Write.vi"("task/channels in"=w443, "data"=w442, "error in"=w447) -> ("task out"=w446:refnum<k21>, "error out"=w444:errorcluster)  [unwired: 10 in, 1 out]
            }
            n147 = Build Array(FALSE, FALSE, FALSE, FALSE, FALSE, FALSE, FALSE, FALSE) -> (w429:bool[])
            n148 = call-poly <vilib>:"DAQmx Write.vi"("task/channels in"=w425, "data"=0.0, "error in"=w424) -> ("task out"=w423:refnum<k21>, "error out"=w422:errorcluster)  [unwired: 10 in, 1 out]
            n149 = call-poly <vilib>:"DAQmx Write.vi"("task/channels in"=w428, "data"=w429, "error in"=w427) -> ("task out"=w420:refnum<k21>, "error out"=w419:errorcluster)  [unwired: 10 in, 1 out]
          }
          frame 1 {
            n150 = Quotient & Remainder(x=w451, y=2) -> (x-y*floor(x/y)=w450:i32)  [unwired: 1 out]
            n151 = case shown="0, Default" w450 {
              tunnel: [w481 w483] -> w454
              tunnel: [w481 w483] -> w453
              tunnel: [w481 TRUE] -> w452
              frame 0, Default {
                w481 = FALSE
                n152 = Wait (ms)(milliseconds to wait=u32 5) -> ()  [unwired: 1 out]
              }
              frame 1 {
                w483 = FALSE
                n153 = Wait (ms)(milliseconds to wait=u32 5) -> ()  [unwired: 1 out]
              }
            }
            "led 2" <- w453
            "led 1" <- w452
            "led 3" <- w454
            n154 = call <vilib>:"Read PNG File.vi"("path to PNG file"=path "F:/CEN 3.2/Dasys/labview project/A_D integration/01.png") -> ("image data"=w456:T1)  [unwired: 8 in, 2 out]
            n155 = call <vilib>:"Draw Flattened Pixmap.vi"("image data"=w456) -> ("new picture"=w455:picture)  [unwired: 8 in]
            n156 = local write "7 Segment"(w455) -> ()
            n157 = for {
              tunnel: [w490] -> w461
              shift-right: [w488] -> w460
              shift-left: w462 -> [w491]
              tunnel: w463 -> [w487]
              tunnel: bool[][] [[FALSE, FALSE, FALSE, FALSE], [FALSE, FALSE, FALSE, FALSE], [FALSE, FALSE, FALSE, FALSE], [FALSE, FALSE, FALSE, FALSE]] -> [w486] mode=indexing
              n158 = local write "Motor:"(w486) -> ()
              n159 = Boolean Array To Number(Boolean array=w486) -> (number=w485:u32)
              n160 = local write "Data to Write"(w485) -> ()
              n161 = Wait Until Next ms Multiple(millisecond multiple=5) -> ()  [unwired: 1 out]
              n162 = call-poly <vilib>:"DAQmx Write.vi"("task/channels in"=w487, "data"=w485, "error in"=w491) -> ("task out"=w490:refnum<k21>, "error out"=w488:errorcluster)  [unwired: 10 in, 1 out]
            }
            n163 = Build Array(TRUE, FALSE, FALSE, FALSE, FALSE, FALSE, FALSE, FALSE) -> (w466:bool[])
            n164 = call-poly <vilib>:"DAQmx Write.vi"("task/channels in"=w476, "data"=1.0, "error in"=w475) -> ("task out"=w478:refnum<k21>, "error out"=w477:errorcluster)  [unwired: 10 in, 1 out]
            n165 = call-poly <vilib>:"DAQmx Write.vi"("task/channels in"=w465, "data"=w466, "error in"=w464) -> ("task out"=w458:refnum<k21>, "error out"=w457:errorcluster)  [unwired: 10 in, 1 out]
          }
          frame 2 {
            n166 = Quotient & Remainder(x=w495, y=2) -> (x-y*floor(x/y)=w494:i32)  [unwired: 1 out]
            n167 = case shown="1" w494 {
              tunnel: [w525 w528] -> w498
              tunnel: [w525 w528] -> w497
              tunnel: [w525 FALSE] -> w496
              frame 0, Default {
                w525 = FALSE
                n168 = Wait (ms)(milliseconds to wait=u32 5) -> ()  [unwired: 1 out]
              }
              frame 1 {
                w528 = TRUE
                n169 = Wait (ms)(milliseconds to wait=u32 5) -> ()  [unwired: 1 out]
              }
            }
            n170 = call <vilib>:"Read PNG File.vi"("path to PNG file"=path "F:/CEN 3.2/Dasys/labview project/A_D integration/02.png") -> ("image data"=w500:T1)  [unwired: 8 in, 2 out]
            n171 = call <vilib>:"Draw Flattened Pixmap.vi"("image data"=w500) -> ("new picture"=w499:picture)  [unwired: 8 in]
            n172 = local write "7 Segment"(w499) -> ()
            n173 = for {
              tunnel: [w534] -> w505
              shift-right: [w532] -> w504
              shift-left: w507 -> [w535]
              tunnel: w506 -> [w531]
              tunnel: bool[][] [[FALSE, FALSE, FALSE, TRUE], [FALSE, FALSE, TRUE, FALSE], [FALSE, TRUE, FALSE, FALSE], [TRUE, FALSE, FALSE, FALSE]] -> [w529] mode=indexing
              n174 = local write "Motor:"(w529) -> ()
              n175 = Boolean Array To Number(Boolean array=w529) -> (number=w530:u32)
              n176 = local write "Data to Write"(w530) -> ()
              n177 = Wait Until Next ms Multiple(millisecond multiple=5) -> ()  [unwired: 1 out]
              n178 = call-poly <vilib>:"DAQmx Write.vi"("task/channels in"=w531, "data"=w530, "error in"=w535) -> ("task out"=w534:refnum<k21>, "error out"=w532:errorcluster)  [unwired: 10 in, 1 out]
            }
            n179 = local write "led 1"(w498) -> ()
            n180 = local write "led 2"(w497) -> ()
            n181 = local write "led 3"(w496) -> ()
            n182 = Build Array(FALSE ("element"), TRUE, FALSE, FALSE, FALSE, FALSE, FALSE, FALSE) -> (w511:bool[])
            n183 = call-poly <vilib>:"DAQmx Write.vi"("task/channels in"=w520, "data"=2.0, "error in"=w519) -> ("task out"=w522:refnum<k21>, "error out"=w521:errorcluster)  [unwired: 10 in, 1 out]
            n184 = call-poly <vilib>:"DAQmx Write.vi"("task/channels in"=w509, "data"=w511, "error in"=w510) -> ("task out"=w502:refnum<k21>, "error out"=w501:errorcluster)  [unwired: 10 in, 1 out]
          }
          frame 3 {
            n185 = Quotient & Remainder(x=w539, y=2) -> (x-y*floor(x/y)=w538:i32)  [unwired: 1 out]
            n186 = case shown="1" w538 {
              tunnel: [w569 w571] -> w542
              tunnel: [w569 w571] -> w541
              tunnel: [w569 w571] -> w540
              frame 0, Default {
                w569 = FALSE
                n187 = Wait (ms)(milliseconds to wait=u32 5) -> ()  [unwired: 1 out]
              }
              frame 1 {
                w571 = TRUE
                n188 = Wait (ms)(milliseconds to wait=u32 5) -> ()  [unwired: 1 out]
              }
            }
            n189 = call <vilib>:"Read PNG File.vi"("path to PNG file"=path "F:/CEN 3.2/Dasys/labview project/A_D integration/03.png") -> ("image data"=w544:T1)  [unwired: 8 in, 2 out]
            n190 = call <vilib>:"Draw Flattened Pixmap.vi"("image data"=w544) -> ("new picture"=w543:picture)  [unwired: 8 in]
            n191 = local write "7 Segment"(w543) -> ()
            n192 = for {
              tunnel: [w577] -> w548
              shift-right: [w575] -> w547
              shift-left: w549 -> [w578]
              tunnel: w550 -> [w574]
              tunnel: bool[][] [[TRUE, FALSE, FALSE, FALSE], [FALSE, TRUE, FALSE, FALSE], [FALSE, FALSE, TRUE, FALSE], [FALSE, FALSE, FALSE, TRUE]] -> [w572] mode=indexing
              n193 = Boolean Array To Number(Boolean array=w572) -> (number=w573:u32)
              "Data to Write" <- w573
              n194 = Wait Until Next ms Multiple(millisecond multiple=5) -> ()  [unwired: 1 out]
              n195 = call-poly <vilib>:"DAQmx Write.vi"("task/channels in"=w574, "data"=w573, "error in"=w578) -> ("task out"=w577:refnum<k21>, "error out"=w575:errorcluster)  [unwired: 10 in, 1 out]
              "Motor:" <- w572
            }
            n196 = local write "led 3"(w540) -> ()
            n197 = local write "led 1"(w542) -> ()
            n198 = local write "led 2"(w541) -> ()
            n199 = Build Array(TRUE, TRUE, FALSE, FALSE, FALSE, FALSE, FALSE, FALSE) -> (w554:bool[])
            n200 = call-poly <vilib>:"DAQmx Write.vi"("task/channels in"=w564, "data"=3.0, "error in"=w563) -> ("task out"=w566:refnum<k21>, "error out"=w565:errorcluster)  [unwired: 10 in, 1 out]
            n201 = call-poly <vilib>:"DAQmx Write.vi"("task/channels in"=w552, "data"=w554, "error in"=w553) -> ("task out"=w546:refnum<k21>, "error out"=w545:errorcluster)  [unwired: 10 in, 1 out]
          }
        }
      }
    }
    n202 = Get Date/Time String(date format (0)=enum16{"short", "long", "abbreviated"}."abbreviated", want seconds? (F)=FALSE) -> (date string=→"Date:":string, time string=→"Time:":string)  [unwired: 1 in]
    n203 = Or(x=w76, y="?") -> (x .or. y?=w67:bool)
  }
  n204 = call <vilib>:"DAQmx Stop Task.vi"("task/channels in"=w10, "error in"=w9) -> ("error out"=w18:errorcluster)  [unwired: 12 in, 1 out]
  n205 = call <vilib>:"DAQmx Stop Task.vi"("task/channels in"=w8, "error in"=w7) -> ("error out"=w16:errorcluster)  [unwired: 12 in, 1 out]
  n206 = call <vilib>:"DAQmx Stop Task.vi"("task/channels in"=w2, "error in"=w1) -> ("error out"=w17:errorcluster)  [unwired: 12 in, 1 out]
  n207 = call <vilib>:"DAQmx Stop Task.vi"("task/channels in"=w6, "error in"=w5) -> ("error out"=w15:errorcluster)  [unwired: 12 in, 1 out]
  n208 = call <vilib>:"DAQmx Stop Task.vi"("task/channels in"=w4, "error in"=w3) -> ("task out"=w13:refnum<k21>, "error out"=w12:errorcluster)  [unwired: 12 in]
  n209 = call <vilib>:"DAQmx Clear Task.vi"("task in"=w13, "error in"=w12) -> ("error out"=w11:errorcluster)  [unwired: 13 in]
  n210 = Merge Errors(w18, w17, w16, w15, w11) -> (w14:errorcluster)
  n211 = call <vilib>:"Simple Error Handler.vi"("error in (no error)"=w14) -> ()  [unwired: 4 in, 5 out]
